vi "Snpshot_Example.vi"(8 "error in (no error)":errorcluster, 11 "handle":i32) -> (0 "error out":errorcluster, 2 "snapshot":picture, 3 "handle out":i32)   [LabVIEW 2021]
uses:
  User32.WebCam_WM_Events.ctl
  <vilib>/picture/picture.llb/imagedata.ctl
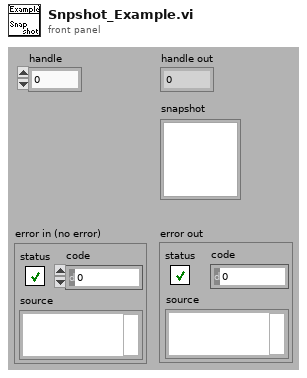
[diagram p1: front panel]
types:
  T1 = typedef "imagedata.ctl" = cluster{"image type":i32, "image depth":i32, "image":u8[], "mask":u8[], "colors":u32[], "Rectangle":cluster{"left":i16, "top":i16, "right":i16, "bottom":i16}}
  T2 = typedef "User32.WebCam_WM_Events.ctl" = i32
  T3 = typedef "LVRectTypeDef.ctl" = cluster{"Left":i16, "Top":i16, "Right":i16, "Bottom":i16}
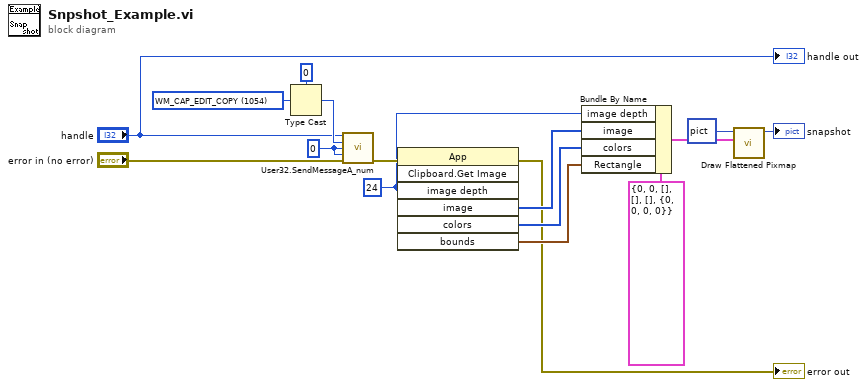
[diagram p0: block diagram]
diagram:
  w5 = 24 ("image depth")
  w2 = T2 1054 items=["WM_CAP_DRIVER_CONNECT"=1034, "WM_CAP_DRIVER_DISCONNECT"=1035, "WM_CAP_EDIT_COPY"=1054, "WM_CAP_SEQUENCE"=1086, "WM_CAP_FILE_SAVEAS"=1047, "WM_CAP_SET_SCALE"=1077, "WM_CAP_SET_PREVIEWRATE"=1076, "WM_CAP_SET_PREVIEW"=1074, "WM_CAP_SET_OVERLAY"=1075, "WM_CAP_FILE_SAVEDIB"=1049] ("Ring")
  w14 = 0 ("wParam")
  n1 = Type Cast(type=0 ("wParam"), x=w2) -> (*(type *) &x=w16:i32)
  n2 = call "User32.SendMessageA_num.vi"("hWnd"="handle", "Msg"=w16, "wParam"=w14, "lParam"=w14, "error in (no error)"="error in (no error)") -> ("error out"=w11:errorcluster)  [unwired: 9 in, 1 out]
  n3 = invoke class="App" method="Clipboard.Get Image"(error in=w11, "image depth"=w5) -> (error out=→"error out":errorcluster, "image"=w8:u8[], "colors"=w7:u32[], "bounds"=w6:T3)  [unwired: 5 in, 3 out]
  n4 = Bundle By Name(cluster=T1 {"image type"=0, "image depth"=0, "image"=[], "mask"=[], "colors"=[], "Rectangle"={"left"=0, "top"=0, "right"=0, "bottom"=0}} ("image data"), "image depth"=w5, "image"=w8, "colors"=w7, "Rectangle"=w6) -> (w9:T1)
  n5 = call <vilib>:"Draw Flattened Pixmap.vi"("image data"=w9, "picture"=picture data[5B]) -> ("new picture"=→"snapshot":picture)  [unwired: 7 in]
  "handle out" <- "handle"
